vi "Get ctrl Secondary axis.vi"(3 "Axis Actions Secondary":T1(ring)) -> (0 "Axis Secondary":dbl)   [LabVIEW 2014]
uses:
  SRE Enum.ctl
  Support Code/Robot Global Data.vi
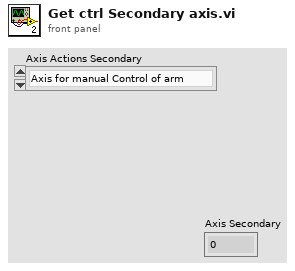
[diagram p1: front panel]
types:
  T1 = enum16{"Axis for manual Control of arm", "Axis for manual Control of Claw", "Rotate Claw"}
  T2 = typedef "SRE Enum.ctl" = enum16{"Start", "Run", "End"}
  T3 = enum16{"Left X", "Left Y", "Left trigger", "R trigger", "R X", "R Y"}[]
  T4 = enum16{"Left X", "Left Y", "Left trigger", "R trigger", "R X", "R Y"}
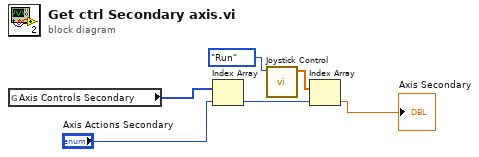
[diagram p0: block diagram]
diagram:
  n1 = global read "Robot Global Data.vi" "Axis Controls Secondary"() -> (w2:T3)
  n2 = Index Array(array=w2, index="Axis Actions Secondary") -> (element=w4:T4)
  n3 = call "Joystick Control.vi"("Enum"=SRE_Enum."Run") -> ("Axis Output PJ"=w6:dbl[])  [unwired: 3 in, 5 out]
  n4 = Index Array(array=w6, index=w4) -> (element=→"Axis Secondary":dbl)
